vi "Save Resource File.vi"(8 "error in (no error)":errorcluster, 9 "Path":path, 10 "File type":string, 11 "Resources":T1) -> (0 "error out":errorcluster)   [LabVIEW 2023]
uses:
  CTLs/Resource Array.ctl
  CTLs/Resource.ctl
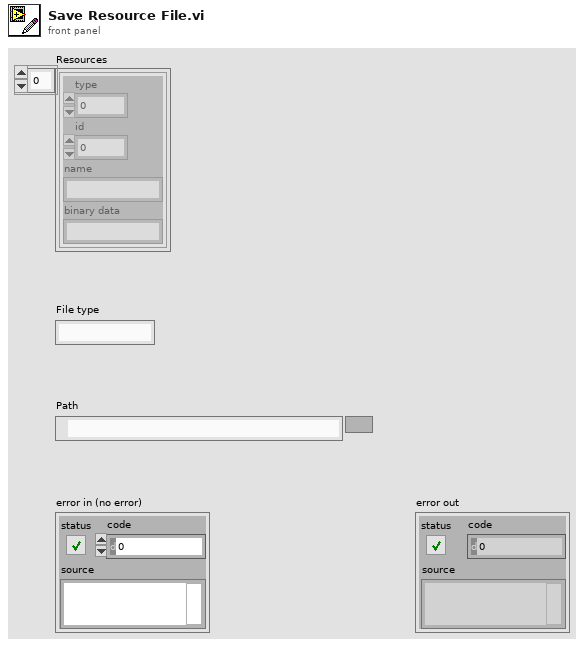
[diagram p1: front panel]
types:
  T1 = typedef "Resource Array.ctl" = T2[]
  T2 = typedef "Resource.ctl" = cluster{"type":u32, "id":i32, "name":string, "binary data":string}
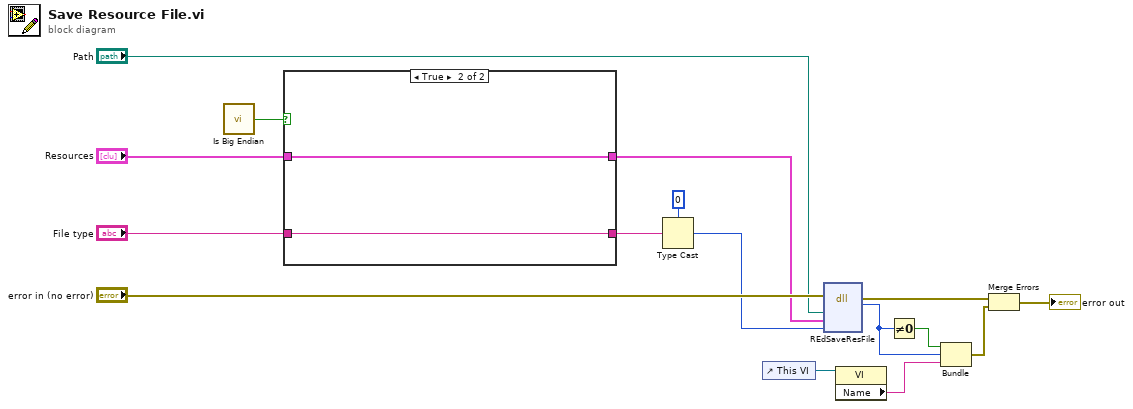
[diagram p0: block diagram]
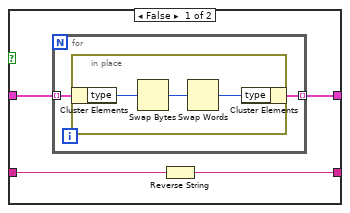
[diagram p2: hidden frame]
diagram:
  n1 = call "Is Big Endian.vi"() -> ("big endian"=w4:bool)
  n2 = case shown="True" w4 {
    tunnel: "Resources" -> [w17 w27]
    tunnel: [w20 w27] -> w7
    tunnel: "File type" -> [w19 w26]
    tunnel: [w18 w26] -> w5
    frame False {
      n3 = for {
        tunnel: [w22] -> w20 mode=indexing
        tunnel: w17 -> [w21] mode=indexing
        n4 = in-place {
          n5 = in-place-cluster #1(w21) -> ("type"=w25:u32)
          n6 = Swap Bytes(anything=w25) -> (byte swapped=w24:u32)
          n7 = Swap Words(1:w24) -> (0:w23:u32)
          n8 = in-place-cluster #1("type"=w23) -> (w22:T2)
        }
      }
      n9 = Reverse String(1:w19) -> (0:w18:string)
    }
    frame True {
    }
  }
  n10 = Type Cast(type=0, x=w5) -> (*(type *) &x=w14:i32)
  n11 = control-ref of="This VI"() -> (w12:refnum<vi>)
  n12 = dll-call lib="LabVIEW" fn="REdSaveResFile"(error in="error in (no error)", "resource binary file"="Path", "resources in"=w7, w14) -> (error out=w2:errorcluster, w10:i32)  [unwired: 5 in, 1 out]
  n13 = property class="VI"(reference=w12) -> ("Name"=w9:string)  [unwired: 1 in, 2 out]
  n14 = Not Equal To 0?(x=w10) -> (x != 0?=w11:bool)
  n15 = Bundle(w11, w10, "Name"=w9) -> (w3:cluster{bool, i32, "Name":string})  [unwired: 1 in]
  n16 = Merge Errors(w2, w3) -> (→"error out":errorcluster)
